vi "Raw_Table_SubarraySel_v1.vi"(2 "error in (no error)":errorcluster, 3 "Column Index":i32, 4 "String to compare":string[](array[string]), 5 "Raw Bar Table Data":string[][](array[string])) -> (0 "error out":errorcluster, 1 "Selected Output":string[][](array[string]))   [LabVIEW 2017]
panel:
  # "v1 can compare 1D string array instead of single string"
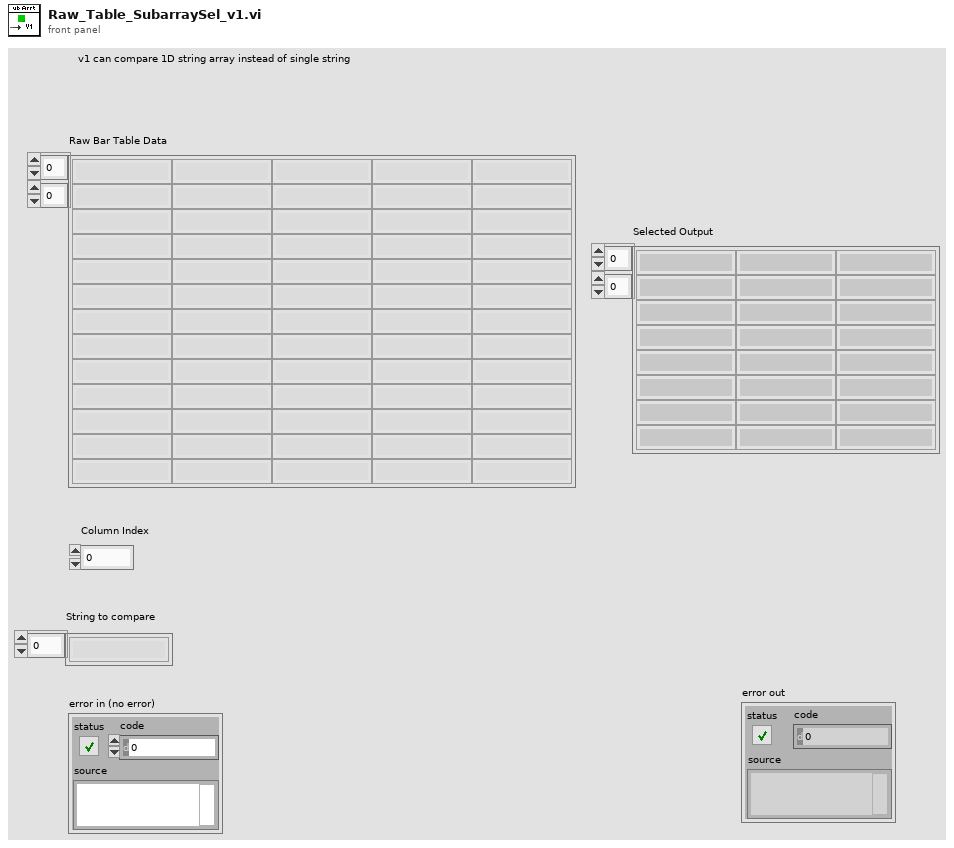
[diagram p1: front panel]
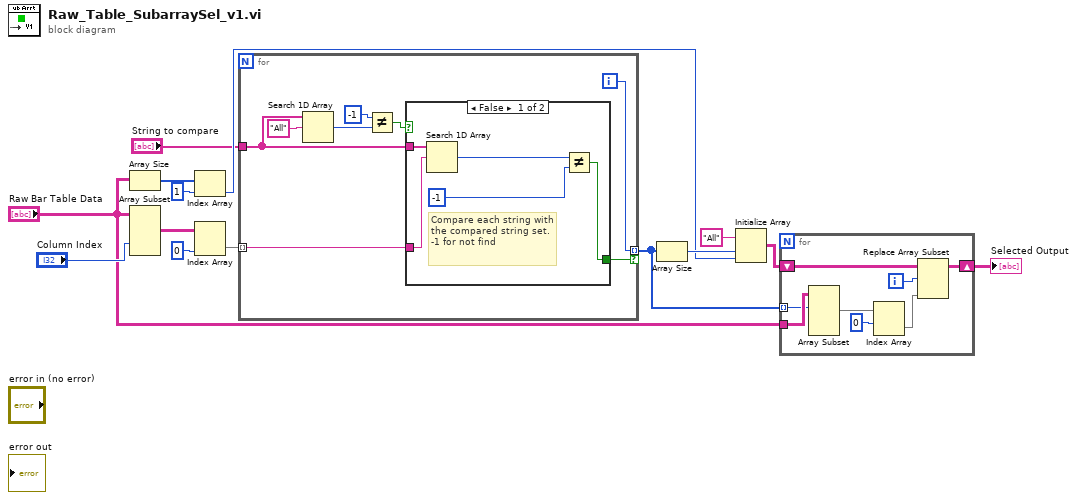
[diagram p0: block diagram]
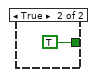
[diagram p2: hidden frame]
diagram:
  n1 = Array Size(array="Raw Bar Table Data") -> (size(s)=w9:i32[])
  n2 = Array Subset(array="Raw Bar Table Data", index (col)="Column Index") -> (w5:string[][])  [unwired: 3 in]
  n3 = Index Array(array=w9, index=1) -> (element=w7:i32)
  n4 = Index Array(array=w5, index (col)=0 ("disabled index (col)")) -> (element=w10:string[])  [unwired: 1 in]
  n5 = for {
    tunnel: w10 -> [w20] mode=indexing
    tunnel: "String to compare" -> [w19]
    tunnel: [w22] -> w12 mode=indexing if=w17
    i -> [w22]
    n6 = Search 1D Array(1D array=w19, element="All") -> (index of element=w18:i32)  [unwired: 1 in]
    n7 = Not Equal?(x=-1, y=w18) -> (x != y?=w21:bool)
    n8 = case shown="False" w21 {
      tunnel: w20 -> [w26 _]
      tunnel: w19 -> [w27 _]
      tunnel: [w25 TRUE] -> w17
      frame False {
        # "Compare each string with the compared string set. -1 for not find"
        n9 = Search 1D Array(1D array=w27, element=w26) -> (index of element=w24:i32)  [unwired: 1 in]
        n10 = Not Equal?(x=w24, y=-1) -> (x != y?=w25:bool)
      }
      frame True {
      }
    }
  }
  n11 = Array Size(array=w12) -> (size(s)=w11:i32)
  n12 = Initialize Array("All", w11, w7) -> (w6:string[][])
  n13 = for {
    tunnel: "Raw Bar Table Data" -> [w36]
    tunnel: w12 -> [w35] mode=indexing
    shift-right: [w32] -> w4
    shift-left: w6 -> [w33]
    i -> [w34]
    n14 = Array Subset(array=w36, index (row)=w35) -> (w31:string[][])  [unwired: 3 in]
    n15 = Index Array(array=w31, index (row)=0) -> (element=w29:string[])  [unwired: 1 in]
    n16 = Replace Array Subset(array=w33, new element=w29, index (row)=w34) -> (w32:string[][])  [unwired: 1 in]
  }
  "Selected Output" <- w4
